vi "myRIO_BRig_RT_dataBlock_nTrials__L.vi"() -> (2 "output_nTrials__L":i32)   [LabVIEW 2014]
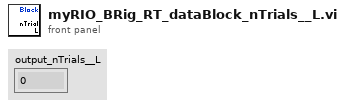
[diagram p1: front panel]
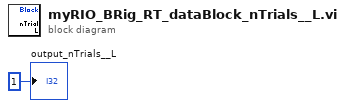
[diagram p0: block diagram]
diagram:
  "output_nTrials__L" <- 1 ("output_iBlock")
